vi "IRISS V2 Teleoperation.vi"() -> ()   [LabVIEW 2016]
uses:
  <vilib>/Math Plots/3D Math Plots/3D Scatter/3D Scatter XCtrl/3D Scatter.xctl
  <vilib>/Analysis/Matrix/Datatypes/RealMatrix.ctl
  Subsystems/Global Variables.vi
  <vilib>/Utility/file.llb/Read Delimited Spreadsheet (DBL).vi
  <vilib>/Math Plots/3D Math Plots/3D Scatter/3D Scatter Datatype/Public/Plot Helper (Vector).vi
  Library/mjglib/var_OCTzHomeDir.vi
  <vilib>/Math Plots/3D Math Plots/3D Plot/3D Plot Datatype/3D Plot Datatype.lvclass
  <vilib>/Analysis/Matrix/NI_Matrix.lvlib
  Functions/EyeRobotDLL.dll
  Library/KevinLibraryAll/labview2011/kevLib2011.lvlib
  <vilib>/Math Plots/3D Math Plots/3D Scatter/3D Scatter Datatype/3D Scatter Datatype.lvclass
panel:
  in  "MS/Auto":bool
  in  "Calib Params?":bool
  in  "Incision":bool caption="To M/S"
  in  "OCT Z PID Gains":cluster{"Kp":dbl, "Kd":dbl, "Ki":dbl}={"Kp"=0.0003, "Kd"=0.0001, "Ki"=0.01}
  out "deltaRoll":sgl
  out "deltaXYZ":sgl[](array[numeric])
  in  "To Regulation":bool
  in  "IRISS GUI":T1(tab)
  in  "U/S Power [%]":sgl min=0 max=100 step=10
  in  "Vac Cmd [mmHg]":sgl min=0 max=600 step=50
  in  "Red Round Box":u32(colorbox)=16711690
  in  "Blue Round Box":u32(colorbox)=16860
  in  "Black Round Box":u32(colorbox)
  out "Vacuum Force [mmHg]  2":i32 caption="[mmHg]"
  in  "IV Height [mmHg]":dbl=30.0 min=0.0 max=90.0 step=10.0
  in  "Irrigation":bool
  in  "Reroute Hold [sec]":dbl=10.0 caption="Hold [sec]"
  in  "Refractive Index":dbl=1.35
  out "Asgn Pt Out of Bound":bool caption="Assign Pt OOB"
  out "Emergency alarm":bool
  out "Remote sender engaged":bool
  out "State changing":bool
  out "Current Run No.":u8
  out "Tip out Posit":dbl[](array[numeric]) caption="Position [mm]" format="%#.3f"
  out "Tip cmd Posit":dbl[](array[numeric]) caption="Command [mm]" format="%#.3f"
  out "State Flag Array":bool[](array[boolean])
  out "Timer":i32 format="%<%M:%S>t"
  in  "Go to Assign Pt":bool
  out "Irrigation Engaged?":bool caption="Irrigation Engaged"
  out "Robot XYZ":refnum<class "3D Plot Datatype.lvclass">[](xcontrol)
  out "Current System State":T2(ring)
  in  "Tracking Mode":u16(ring) items=["Joint Mode", "XYZ Mode"]
  in  "Stage Z [mm]":dbl=100.0 min=-120.0 max=120.0 step=0.5
  in  "Stage Y [mm]":dbl=70.0 min=-120.0 max=100.0 step=0.5
  in  "Gripper":dbl
  in  "OCT Cmd Z [mm]":dbl min=-25.0 max=14.0 step=0.5
  out "Joint Out":dbl[](array[numeric])
  out "Robot Status Array":bool[](array[boolean])
  in  "L1 [deg]":dbl=-40.0
  in  "L2 [deg]":dbl=15.0
  in  "L3 [mm]":dbl=-5.0 step=0.1
  out "Status 2":bool[](array[boolean])
  in  "L4 [deg]":dbl=-10.0 step=0.1
  in  "Home":bool
  out "OCT Z out [mm]":dbl caption="OCT Out Z [mm]" format="%#.4f"
  in  "Tool Type":i32=6
  in  "Tool Offset [mm]":dbl=-50.68
  out "Grasp out":dbl format="%#.4g"
  in  "OCTz Home Dir":bool
  in  "Remote Control Source":u16(ring) caption="Remote Source" items=["None", "Surgical Console", "Joystick", "Rigid Joystick", "Zeiss PC", "MJG C++ Teleoperation", "A-Scan", ""]
  in  "Reset Joystick":bool caption="Encoder Reset"
  out "Send Count":u64
  out "Receive Count":u64
  out "Arm ID Ind":i32
  out "Status":bool
  in  "Stage X [mm]":dbl=30.0 min=-120.0 max=120.0 step=0.5
  out "XYZ Stage out":dbl[](array[numeric])
  out "XYZ Stage cmd":dbl[](array[numeric])
  out "DH Params":cluster{"d_DH":dbl[][], "ty":dbl[][]}
  in  "Eye No":i16=1 min=1 step=1
  in  "Reroute Transit Vacf":dbl=100.0
  in  "Z Rot Axis":dbl=1.0
  in  "Z Dist Thld":dbl[](array[numeric])=[3.0, 5.0] caption="Z Distance Threshould"
  in  "Vac Extremum":dbl[](array[numeric])=[68.0, 68.0] caption="Vacuum Extremum"
  out "Value [mmHg]":i8
  in  "Save Data":bool
  out "File Exists":bool
  out "File Path":path
  out "Elaspsed Time [s]":sgl
  in  "Data No":i16=1 min=1 step=1
  in  "Total Time":i16=90 min=1 step=1
  in  "Min PC Gap":dbl=0.1 caption="Min PC Gap [mm]" min=0.0 max=10.0 step=0.1 format="%#.3g"
  in  "Min AC Gap":dbl=0.1 caption="Min AC Gap [mm]" min=0.0 max=10.0 step=0.1 format="%#.3g"
  in  "Joint Limits":dbl[][](array[numeric])=[[-68.0, -4.0], [-26.0, 52.0], [-40.0, 23.0], [-180.0, 180.0]] format="%#.3g"
  out "L4 Waveform Graph":dbl[](graph)
  out "L3 Waveform Graph":dbl[](graph)
  out "L2 Waveform Graph":dbl[](graph)
  out "L1 Waveform Graph":dbl[](graph)
  in  "Inc Ctrl":dbl[](array[numeric])=[0.1, 0.05, 0.05] caption="Increment Control"
  out "Stage command":dbl[](array[numeric])
  in  "Vscan path":path=path "D:/IRISSoft LV2016 beta/Host Demo/ThorlabsData/Eye1/VSCAN_0002.raw"
  in  "size_xyz_mm":dbl[](array[numeric])=[16.0, 16.0, 9.4, 1.0]
  in  "size_xyz":dbl[](array[numeric])=[400.0, 400.0, 1024.0, 1.0]
  in  "Confirm":bool
  in  "Image index":i32=200
  out "O":dbl[](array[numeric])
  out "New TOI":dbl[][](array[numeric])
  out "Original TOI":dbl[][](array[numeric])
  in  "Stop Accurus":bool caption="To M/S"
  in  "L3 Go Home":bool caption="To M/S"
  in  "Program Stop":bool
  # "M/S\n \nAuto"
  # "Tool Tip Location"
  # "Tracking Planning"
  # "RCM"
  # "X\nY\nZ"
  # "X\nY\nZ"
  # "Tool"
  # "Trajectory"
  # "System Progress"
  # "Assign Point Rerouting"
  # "Trajectory Generation"
  # "X\nY\nZ"
  # "X Offset"
  # "Y Offset"
  # "Homing finished"
  # "Z Offset"
  # "M/S initialization finished"
  # "Tool Cruising Boundaries"
  # "XY-plane"
  # "Trajecoty loading finished"
  # "Aiming finished"
  # "Tool engaged"
  # "Z-axis"
  # "Phaco Machine"
  # "Tracking initialization finished"
  # "In Tracking"
  # "Rerouting finished"
  # "X\nY"
  # "X\nY"
  # "In regulation"
  # "Robot Control"
  # "Homing"
  # "Joint Definition"
  # "Arm"
  # "Tool"
  # "Stage"
  # "Robot Status"
  # "Joint M/S Cmd"
  # "HARDWARE_NOT_PRESENT"
  # "HARDWARE_NOT_FOUND_ALL_DRIVES"
  # "HARDWARE_SENSOR_FAULT"
  # "NOT_RUNNING"
  # "COMMUNICATION_ERROR"
  # "KINEMATICS_NO_SOLUTION"
  # "OCT Control"
  # "KINEMATICS_INSERTION_LENGTH_TOO_SMALL"
  # "COMMAND_BEYOND_JOINT_RANGE"
  # "COMMAND_TOO_LARGE"
  # "Irrigation and Aspiration"
  # "IOP Control"
  # "Data Saving"
  # "Irrigation"
  # "Aspiration"
  # "ACh"
  # "Vitreous"
  # "Rotation & Vacuum Force Scheduling"
  # "Joint Motion & Control"
  # "Space Deform Parameters"
  # "Depth Ctrl"
  # "S"
  # "R"
  # "[deg]"
  # "T"
  # "[mm]"
  # "First Track Point"
  # "AC & PC Gap"
  # "X1"
  # "[mm]"
  # "Y"
  # "[mm]"
  # "Z"
  # "[mm]"
  # "L4"
  # "[deg]"
  # "Joint Limits"
  # "Error Message"
  # "Incision"
  # "Min."
  # "Max."
  # "L1"
  # "[deg]"
  # "L1"
  # "L2"
  # "L2"
  # "[deg]"
  # "L3"
  # "[mm]"
  # "L3"
  # "L4"
  # "[deg]"
  # "L4"
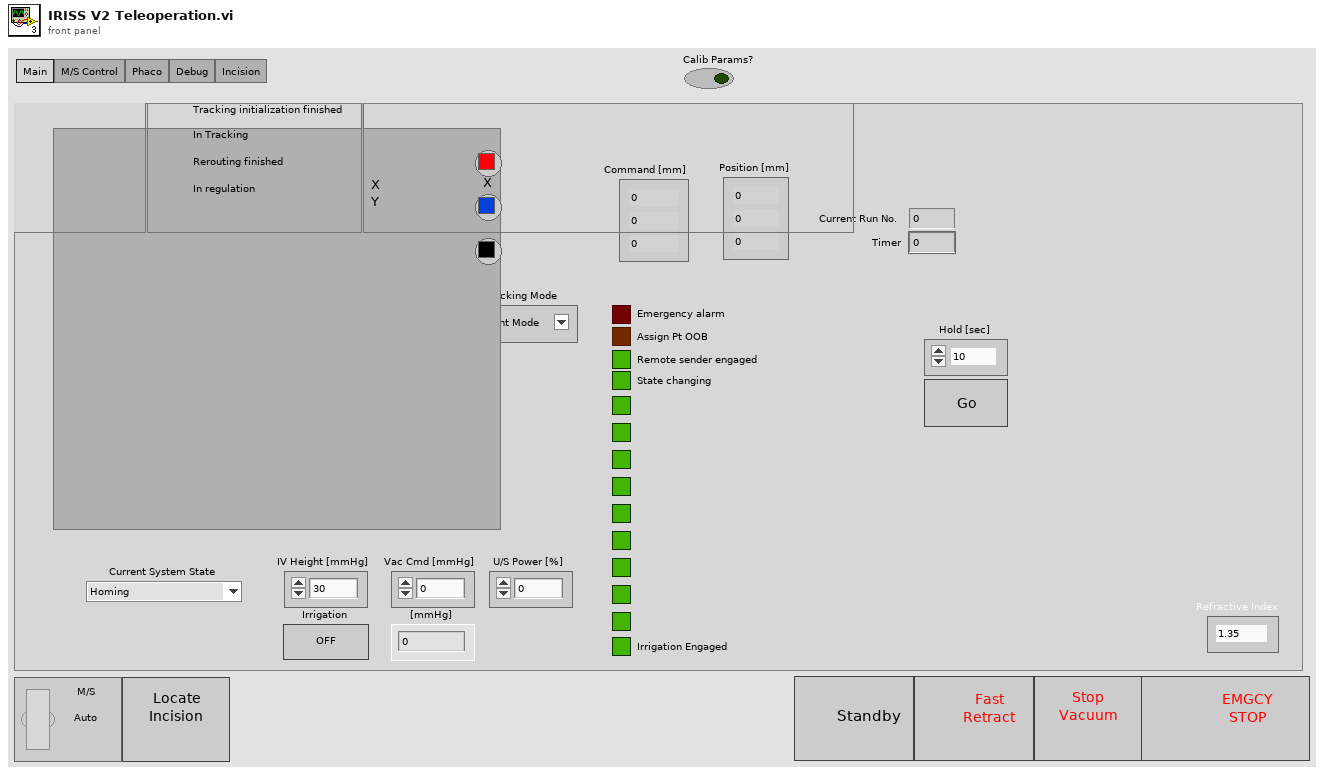
[diagram p1: front panel]
types:
  T1 = enum32{"Main", "M/S Control", "Phaco", "Debug", "Incision"}
  T2 = enum16{"Homing", "M/S Initialization", "M/S Operation", "Aiming", "Engaging", "Trajectory Loading", "Tracking Initialization", "Tracking", "Rerouting", "Regulation"}
  T3 = cluster{"Traj Px Array":dbl[], "Traj Py Array":dbl[], "Traj Pz Array":dbl[], "Speed Array":dbl[], "Depth Array":dbl[], "Traj Joint1 Array":dbl[], "Traj Joint2 Array":dbl[], "Traj Joint3 Array":dbl[], "Traj Joint4 Array":dbl[], "Traj Joint5 Array":dbl[]}
  T4 = typedef "NI_Matrix.lvlib/RealMatrix.ctl" = dbl[][]
  T5 = cluster{"X Grid":dbl[], "Y Grid":dbl[], "Za_true Surf":dbl[][], "Iris Center":dbl[], "Zp_true Surf":dbl[][], "Pinv":T4, "za_true":dbl, "za_work":dbl, "zp_work":dbl, "zp_true":dbl}
  T6 = enum8{"Enabled", "Disabled", "Disabled and Grayed Out"}
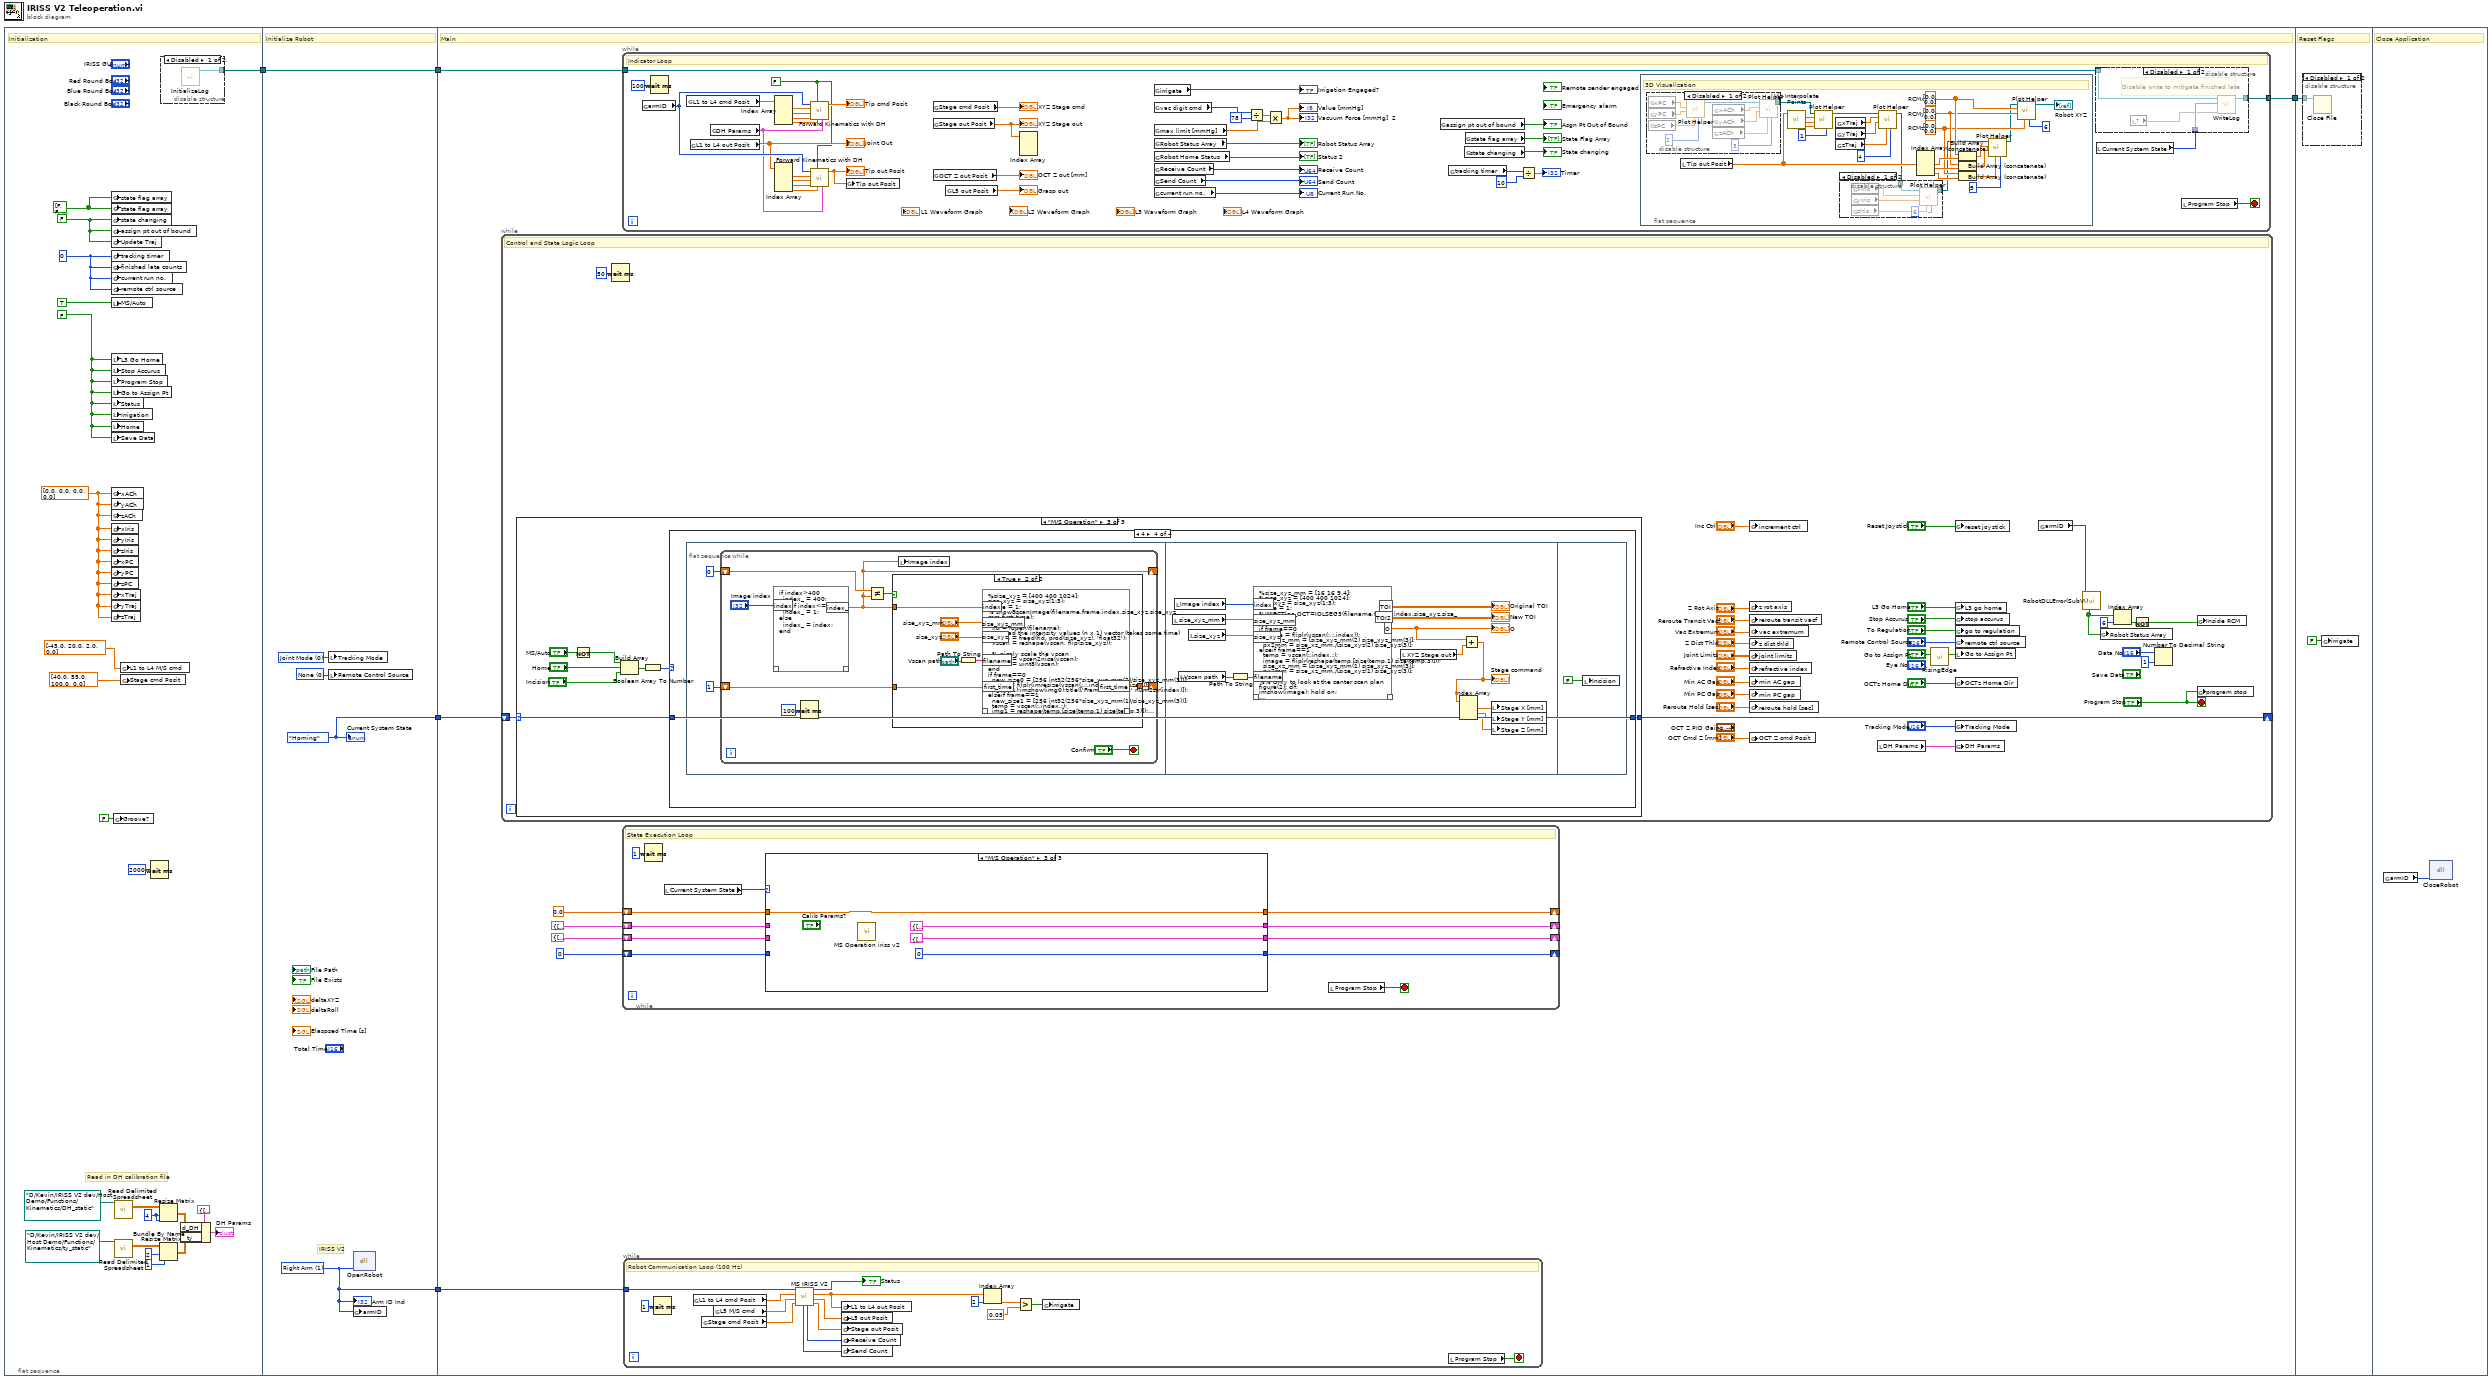
[diagram p0: block diagram]
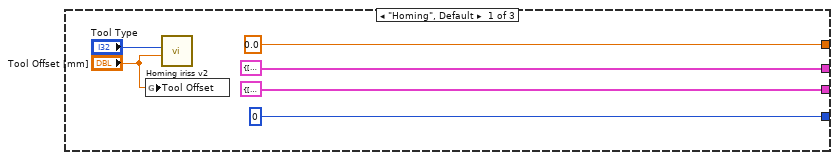
[diagram p3: hidden frame]
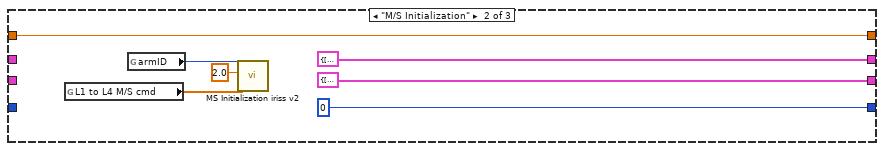
[diagram p4: hidden frame]
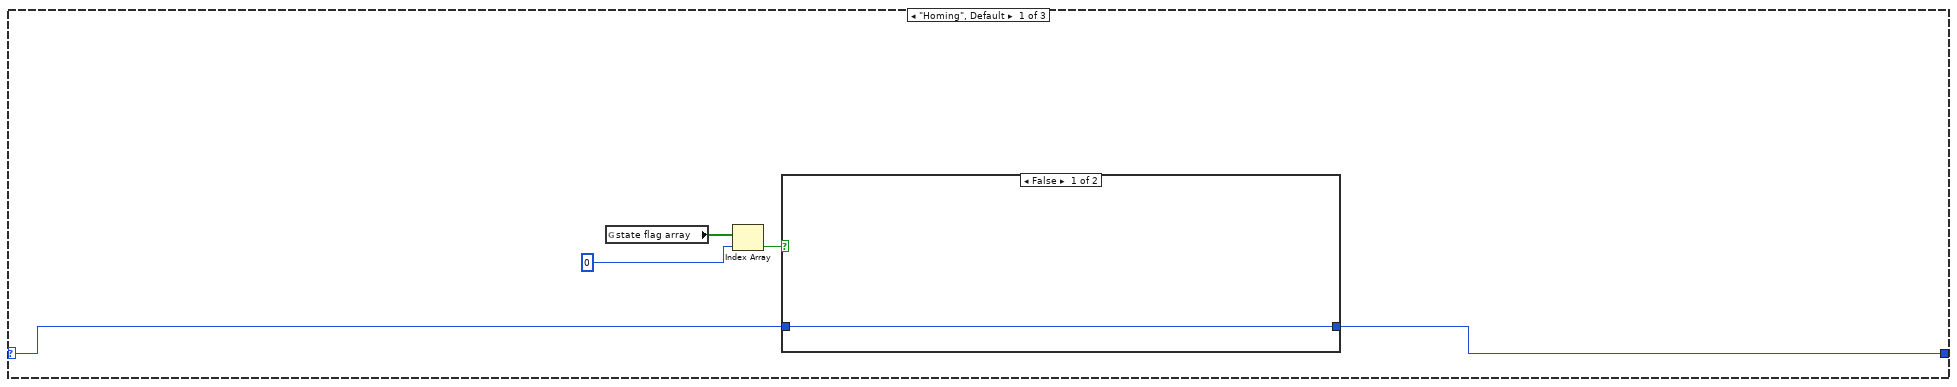
[diagram p8: hidden frame]
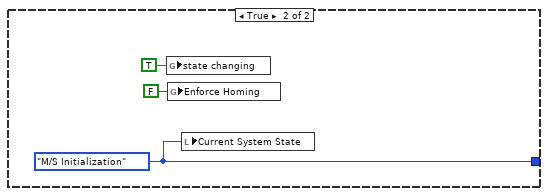
[diagram p9: hidden frame]
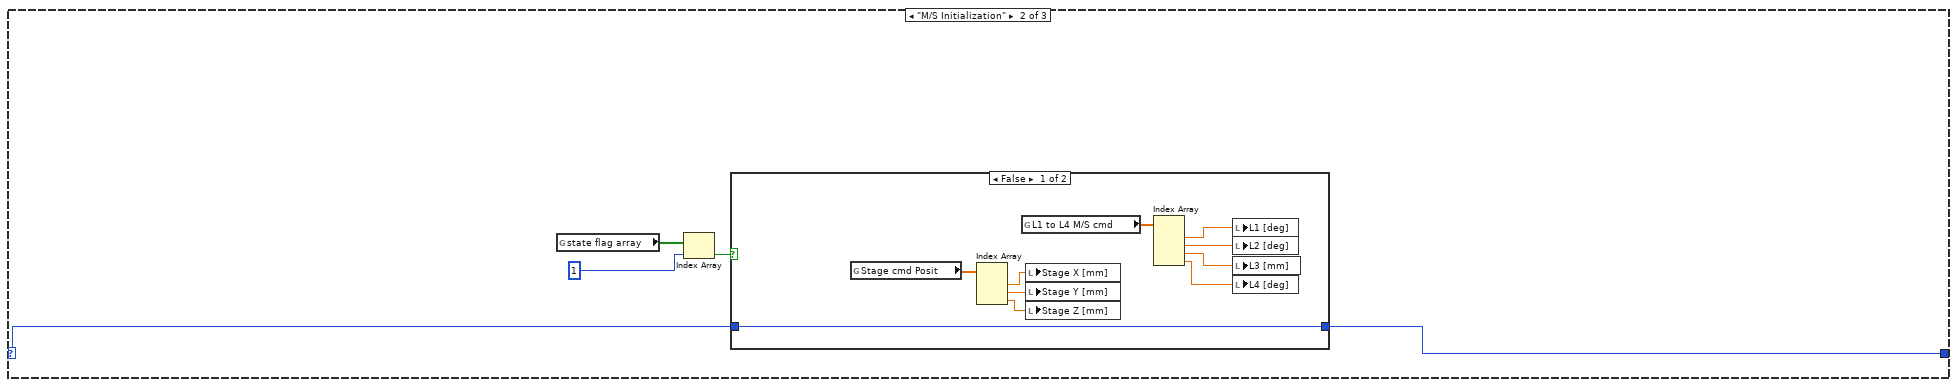
[diagram p10: hidden frame]
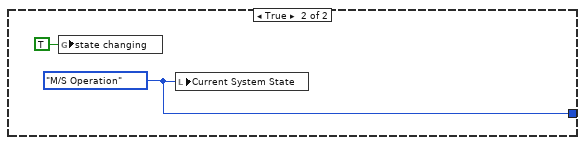
[diagram p11: hidden frame]
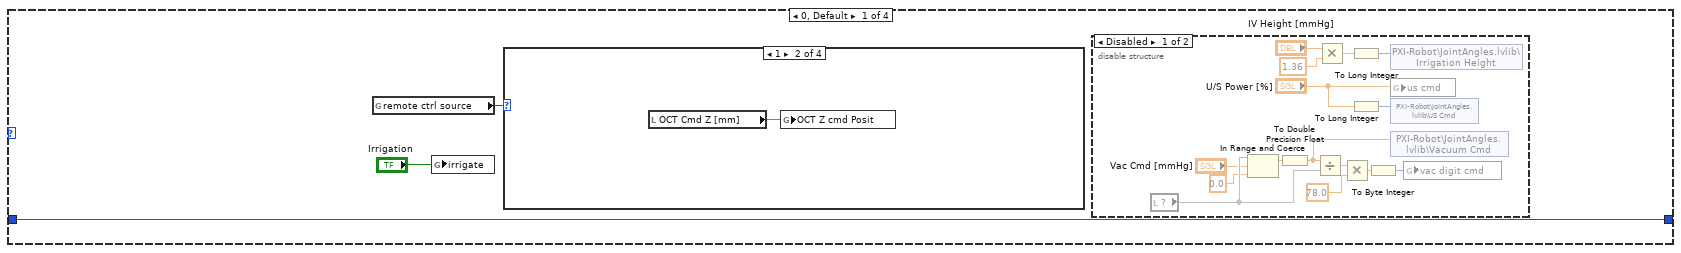
[diagram p12: hidden frame]
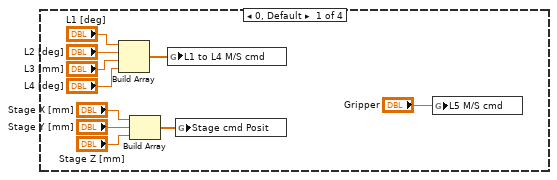
[diagram p14: hidden frame]
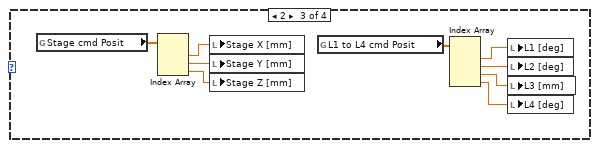
[diagram p15: hidden frame]
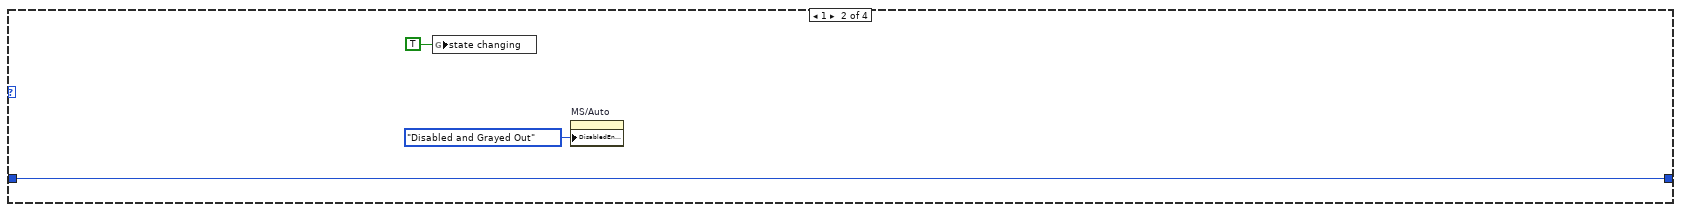
[diagram p17: hidden frame]
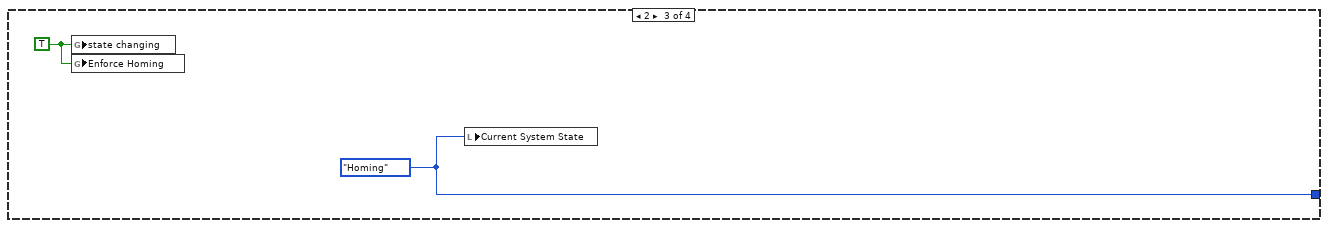
[diagram p18: hidden frame]
diagram:
  n1 = flat-sequence {
    tunnel: [w26] -> w3
    tunnel: [w32] -> w4
    tunnel: w3 -> [w33]
    tunnel: [w33] -> w2
    tunnel: [w30] -> w1
    tunnel: w4 -> [w41]
    tunnel: w2 -> [w40]
    tunnel: [w39] -> w5
    tunnel: w1 -> [w36]
    tunnel: w5 -> [w317]
    frame #0 {
      w14 = 4 ("number of rows")
      w21 = dbl[] [0.0, 0.0, 0.0, 0.0] ("First Trk Pt 2")
      w20 = 0 ("finished late counts")
      w25 = bool[] [FALSE, FALSE, FALSE, FALSE, FALSE, FALSE, FALSE, FALSE, FALSE] ("state flag array")
      w24 = FALSE ("state changing")
      w22 = FALSE ("program stop")
      # "Read in DH calibration file"
      # "Initialization"
      n2 = global write "Global Variables.vi" "state flag array"(w25) -> ()
      n3 = global write "Global Variables.vi" "state flag array"(w25) -> ()
      n4 = global write "Global Variables.vi" "state changing"(w24) -> ()
      n5 = global write "Global Variables.vi" "assign pt out of bound"(w24) -> ()
      n6 = global write "Global Variables.vi" "Update Traj"(w24) -> ()
      n7 = global write "Global Variables.vi" "tracking timer"(w20) -> ()
      n8 = global write "Global Variables.vi" "finished late counts"(w20) -> ()
      n9 = global write "Global Variables.vi" "current run no."(w20) -> ()
      n10 = global write "Global Variables.vi" "remote ctrl source"(w20) -> ()
      n11 = local write "MS/Auto"(TRUE ("MS/Auto")) -> ()
      n12 = local write "L3 Go Home"(w22) -> ()
      n13 = local write "Stop Accurus"(w22) -> ()
      n14 = local write "Program Stop"(w22) -> ()
      n15 = local write "Go to Assign Pt"(w22) -> ()
      n16 = local write "Status"(w22) -> ()
      n17 = local write "Irrigation"(w22) -> ()
      n18 = local write "Home"(w22) -> ()
      n19 = local write "Save Data"(w22) -> ()
      n20 = global write "Global Variables.vi" "xACh"(w21) -> ()
      n21 = global write "Global Variables.vi" "yACh"(w21) -> ()
      n22 = global write "Global Variables.vi" "zACh"(w21) -> ()
      n23 = global write "Global Variables.vi" "xIris"(w21) -> ()
      n24 = global write "Global Variables.vi" "yIris"(w21) -> ()
      n25 = global write "Global Variables.vi" "zIris"(w21) -> ()
      n26 = global write "Global Variables.vi" "xPC"(w21) -> ()
      n27 = global write "Global Variables.vi" "yPC"(w21) -> ()
      n28 = global write "Global Variables.vi" "zPC"(w21) -> ()
      n29 = global write "Global Variables.vi" "xTraj"(w21) -> ()
      n30 = global write "Global Variables.vi" "yTraj"(w21) -> ()
      n31 = global write "Global Variables.vi" "zTraj"(w21) -> ()
      n32 = global write "Global Variables.vi" "Groove?"(FALSE ("Groove?")) -> ()
      n33 = call-poly <vilib>:"Read Delimited Spreadsheet.vi"("file path (dialog if empty)"=path "D:/Kevin/IRISS V2 dev/Host Demo/Functions/Kinematics/DH_static" ("file path (use dialog)")) -> ("all rows"=w15:dbl[][])  [unwired: 9 in, 5 out]
      n34 = call-poly <vilib>:"Read Delimited Spreadsheet.vi"("file path (dialog if empty)"=path "D:/Kevin/IRISS V2 dev/Host Demo/Functions/Kinematics/ty_static" ("file path (use dialog)")) -> ("all rows"=w13:dbl[][])  [unwired: 9 in, 5 out]
      n35 = global write "Global Variables.vi" "L1 to L4 M/S cmd"(dbl[] [-45.0, 20.0, 2.0, 0.0] ("First Trk Pt 2")) -> ()
      n36 = global write "Global Variables.vi" "Stage cmd Posit"(dbl[] [40.0, 55.0, 100.0, 0.0] ("First Trk Pt 2")) -> ()
      n37 = Wait (ms)(milliseconds to wait=u32 2000) -> ()  [unwired: 1 out]
      n38 = Resize Matrix(1:w14, 2:w14, 4:w15) -> (0:w9:dbl[][])
      n39 = Resize Matrix(1:1 ("number of columns"), 2:2 ("number of rows"), 4:w13) -> (0:w8:dbl[][])
      n40 = disable-structure shown="Disabled" {
        disable-tunnel: [w28 _] -> w26
        frame Disabled {
          n41 = call "InitializeLog.vi"() -> ("Byte Stream File out"=w28:refnum<file>)  [unwired: 11 in]
        }
        frame Enabled {
        }
      }
      n42 = Bundle By Name(cluster=cluster{"d_DH":dbl[][], "ty":dbl[][]} {"d_DH"=[[0.0, -0.04858099004841317, 1.1971672750675049, 0.0], [0.0, -1.576475511297109, 0.0, 0.0], [-0.3552491783526254, 0.0, -1.1064589410656984, 0.2058446720735121], [-1.0573457532495087, 1.0278049025155533, 0.011917110633363169, -0.004023577880993236]], "ty"=[[0.04320445582455471], [0.011728642746432275]]} ("input cluster"), "d_DH"=w9, "ty"=w8) -> (→"DH Params":cluster{"d_DH":dbl[][], "ty":dbl[][]})
    }
    frame #1 {
      w29 = u16 0 items=["Joint Mode", "XYZ Mode"] ("Tracking Mode")
      w31 = u16 0 items=["None", "Surgical Console", "Joystick", "MJG Teleoperation", "MJG C++ Teleoperation"] ("Remote Control Source 2")
      w32 = T2."Homing" ("Current State")
      w30 = 1 items=["Left Arm", "Right Arm"] ("Left or Right Arm")
      # "IRISS V2"
      # "Initialize Robot"
      n43 = local write "Tracking Mode"(w29) -> ()
      n44 = local write "Remote Control Source"(w31) -> ()
      n45 = dll-call lib="D:/Kevin/IRISS V2 dev/Host Demo/Functions/EyeRobotDLL.dll" fn="OpenRobot" label="Open"("id"=w30) -> ()  [unwired: 5 in, 2 out]
      n46 = global write "Global Variables.vi" "armID"(w30) -> ()
      "Arm ID Ind" <- w30
      "Current System State" <- w32
    }
    frame #2 {
      # "Main"
      n47 = while {
        shift-right: [w195] -> _
        shift-left: w41 -> [w196]
        stop <- "Program Stop" stop-if-true
        # "Control and State Logic Loop"
        n48 = case shown="\"M/S Operation\"" w196 {
          selector: w196 -> [w208 w215 w239]
          tunnel: [w207 w216 w238] -> w195
          frame "Homing", Default {
            # "State Diagram"
            n49 = global read "Global Variables.vi" "state flag array"() -> (w209:bool[])
            n50 = Index Array(array=w209, index=0) -> (element=w206:bool)
            n51 = case shown="False" w206 {
              tunnel: [w211 w213] -> w207
              tunnel: w208 -> [w211 _]
              frame False {
                # "homing in process"
              }
              frame True {
                w213 = T2."M/S Initialization" ("Current State")
                # "finish homing"
                n52 = global write "Global Variables.vi" "state changing"(TRUE ("state changing")) -> ()
                n53 = global write "Global Variables.vi" "Enforce Homing"(FALSE ("Enforce Homing")) -> ()
                n54 = local write "Current System State"(w213) -> ()
              }
            }
          }
          frame "M/S Initialization" {
            n55 = global read "Global Variables.vi" "state flag array"() -> (w218:bool[])
            n56 = Index Array(array=w218, index=1) -> (element=w217:bool)
            n57 = case shown="False" w217 {
              tunnel: [w229 w230] -> w216
              tunnel: w215 -> [w229 _]
              frame False {
                n58 = global read "Global Variables.vi" "Stage cmd Posit"() -> (w223:dbl[])
                n59 = Index Array(array=w223) -> (element #1=w221:dbl, element #2=w222:dbl, element #3=w220:dbl)  [unwired: 3 in]
                n60 = global read "Global Variables.vi" "L1 to L4 M/S cmd"() -> (w228:dbl[])
                n61 = local write "Stage X [mm]"(w221) -> ()
                n62 = local write "Stage Y [mm]"(w222) -> ()
                n63 = local write "Stage Z [mm]"(w220) -> ()
                n64 = Index Array(array=w228) -> (element #1=w227:dbl, element #2=w226:dbl, element #3=w225:dbl, element #4=w224:dbl)  [unwired: 4 in]
                n65 = local write "L1 [deg]"(w227) -> ()
                n66 = local write "L2 [deg]"(w226) -> ()
                n67 = local write "L3 [mm]"(w225) -> ()
                n68 = local write "L4 [deg]"(w224) -> ()
              }
              frame True {
                w230 = T2."M/S Operation" ("Current State")
                n69 = global write "Global Variables.vi" "state changing"(TRUE ("state changing")) -> ()
                n70 = local write "Current System State"(w230) -> ()
              }
            }
          }
          frame "M/S Operation" {
            n71 = Not(x="MS/Auto") -> (.not. x?=w237:bool)
            n72 = Build Array(w237, "Home", "Incision") -> (w236:bool[])
            n73 = Boolean Array To Number(Boolean array=w236) -> (number=w235:u32)
            n74 = case shown="4" w235 {
              tunnel: w239 -> [w242 w279 _ w283]
              tunnel: [w242 w279 w282 w283] -> w238
              frame 0, Default {
                n75 = global read "Global Variables.vi" "remote ctrl source"() -> (w241:u16)
                n76 = global write "Global Variables.vi" "irrigate"("Irrigation") -> ()
                n77 = case shown="1" w241 {
                  frame 0, Default {
                    n78 = Build Array("L1 [deg]", "L2 [deg]", "L3 [mm]", "L4 [deg]") -> (w258:dbl[])
                    n79 = Build Array("Stage X [mm]", "Stage Y [mm]", "Stage Z [mm]") -> (w263:dbl[])
                    n80 = global write "Global Variables.vi" "L1 to L4 M/S cmd"(w258) -> ()
                    n81 = global write "Global Variables.vi" "Stage cmd Posit"(w263) -> ()
                    n82 = global write "Global Variables.vi" "L5 M/S cmd"("Gripper") -> ()
                  }
                  frame 1 {
                    n83 = local read "OCT Cmd Z [mm]"() -> (w268:dbl)
                    n84 = global write "Global Variables.vi" "OCT Z cmd Posit"(w268) -> ()
                  }
                  frame 2 {
                    n85 = global read "Global Variables.vi" "Stage cmd Posit"() -> (w277:dbl[])
                    n86 = Index Array(array=w277) -> (element #1=w276:dbl, element #2=w275:dbl, element #3=w274:dbl)  [unwired: 3 in]
                    n87 = local write "Stage X [mm]"(w276) -> ()
                    n88 = local write "Stage Y [mm]"(w275) -> ()
                    n89 = local write "Stage Z [mm]"(w274) -> ()
                    n90 = global read "Global Variables.vi" "L1 to L4 cmd Posit"() -> (w269:dbl[])
                    n91 = Index Array(array=w269) -> (element #1=w272:dbl, element #2=w271:dbl, element #3=w270:dbl, element #4=w273:dbl)  [unwired: 4 in]
                    n92 = local write "L1 [deg]"(w272) -> ()
                    n93 = local write "L2 [deg]"(w271) -> ()
                    n94 = local write "L3 [mm]"(w270) -> ()
                    n95 = local write "L4 [deg]"(w273) -> ()
                  }
                  frame 3 {
                  }
                }
                n96 = disable-structure shown="Disabled" {
                  frame Disabled {
                    n97 = local read item#-1() -> (w249)
                    n98 = In Range and Coerce(upper limit=w249, x="Vac Cmd [mmHg]", lower limit=0.0) -> (coerced(x)=w250:dbl)  [unwired: 1 out]
                    n99 = To Double Precision Float(number=w250) -> (double precision float=w251:dbl)
                    n100 = Divide(x=w251, y=w249) -> (x/y=w244:dbl)
                    n101 = Multiply(x="IV Height [mmHg]", y=1.36) -> (x*y=w255:dbl)
                    n102 = Multiply(x=w244, y=78.0) -> (x*y=w246:dbl)
                    n103 = To Long Integer(number=w255) -> (32bit integer=w256:i32)
                    n104 = To Long Integer(number="U/S Power [%]") -> (32bit integer=w252:i32)
                    n105 = To Byte Integer(number=w246) -> (8bit integer=w243:i8)
                    n106 = shared-variable "PXI-Robot\\JointAngles.lvlib\\Irrigation Height"(w256) -> ()  [unwired: 1 in, 1 out]
                    n107 = global write "Global Variables.vi" "us cmd"("U/S Power [%]") -> ()
                    n108 = shared-variable "PXI-Robot\\JointAngles.lvlib\\US Cmd"(w252) -> ()  [unwired: 1 in, 1 out]
                    n109 = shared-variable "PXI-Robot\\JointAngles.lvlib\\Vacuum Cmd"(w251) -> ()  [unwired: 1 in, 1 out]
                    n110 = global write "Global Variables.vi" "vac digit cmd"(w243) -> ()
                  }
                  frame Enabled {
                  }
                }
              }
              frame 1 {
                n111 = global write "Global Variables.vi" "state changing"(TRUE ("state changing")) -> ()
                n112 = property on="MS/Auto" class="Bool (strict)"("DisabledEnum"=T6."Disabled and Grayed Out" ("Disabled")) -> ()  [unwired: 2 in, 2 out]
              }
              frame 2 {
                w282 = T2."Homing" ("Current State")
                w281 = TRUE ("state changing")
                n113 = global write "Global Variables.vi" "state changing"(w281) -> ()
                n114 = global write "Global Variables.vi" "Enforce Homing"(w281) -> ()
                n115 = local write "Current System State"(w282) -> ()
              }
              frame 4 {
                n116 = flat-sequence {
                  frame #0 {
                    n117 = while {
                      shift-right: [w290] -> _
                      shift-left: 0 -> [w291]
                      shift-right: [w288] -> _
                      shift-left: 1 -> [w289]
                      stop <- "Confirm" stop-if-true
                      n118 = script code="if index>400\n  index_ = 400;\nelseif index<=0\n  index_ = 1;\nelse\n  index_ = index;\nend"("index"="Image index") -> ("index_"=w290:dbl)  [unwired: 1 in, 1 out]
                      n119 = Wait (ms)(milliseconds to wait=u32 100) -> ()  [unwired: 1 out]
                      n120 = Not Equal?(x=w291, y=w290) -> (x != y?=w292:bool)
                      n121 = case shown="True" w292 {
                        tunnel: w290 -> [_ w301]
                        tunnel: w289 -> [w294 w299]
                        tunnel: [w294 w298] -> w288
                        frame False {
                        }
                        frame True {
                          n122 = Path To String(path="Vscan path") -> (string=w300:string)
                          n123 = script code="%size_xyz = [400 400 1024];\nsize_xyz = size_xyz(1:3);\nframe = 1;\n% showBscanImage(filename,frame,index,size_xyz,size_xyz_mm,first_time);\nif first_time\n  fid = fopen(filename);\n  % Read the intensity values (n x 1) vector (takes some time)\n  vscan = fread(fid, prod(size_xyz), 'float32');\n  vscan = reshape(vscan, flip(size_xyz));\n\n  % nicely scale the vscan\n  vscan = vscan2nice(vscan);\n  vscan = uint8(vscan);\nend\nif frame==0\n  new_size0 = [256 int32(256*size_xyz_mm(2)/size_xyz_mm(3))];\n  img0 = filplr(imresize(vscan(:,:,index),new_size0));\n  figure(1);imshow(img0);title(['Frame:0 Index:' num2str(index)]);\nelseif frame==1\n  new_size1 = [256 int32(256*size_xyz_mm(1)/size_xyz_mm(3))];\n  temp = vscan(:,index,:);\n  img1 = reshape(temp,[size(temp,1) size(temp,3)]);\n  img1 = fliplr(imresize(img1,new_size1));\n  figure(1);imshow(img1);title(['Frame:1 Index:' num2str(index)]);\nend\n\nfirst_time = 0;"("index"=w301, "size_xyz_mm"="size_xyz_mm", "size_xyz"="size_xyz", "filename"=w300, "first_time"=w299) -> ("first_time"=w298:dbl)  [unwired: 1 in, 1 out]
                        }
                      }
                      n124 = local write "Image index"(w290) -> ()
                    }
                  }
                  frame #1 {
                    n125 = local read "size_xyz_mm"() -> (w313:dbl[])
                    n126 = local read "Image index"() -> (w314:i32)
                    n127 = local read "Vscan path"() -> (w311:path)
                    n128 = local read "size_xyz"() -> (w312:dbl[])
                    n129 = Path To String(path=w311) -> (string=w310:string)
                    n130 = script code="%size_xyz_mm = [16 16 9.4];\n%size_xyz = [400 400 1024];\nsize_xyz = size_xyz(1:3);\nframe = 1;\n%INJECTloc_OCT=IOLSEG3(filename,frame,index,size_xyz,size_xyz_mm);\n\nif frame==0\n  image = fliplr(vscan(:,:,index));\n  size_xz_mm = [size_xyz_mm(2) size_xyz_mm(3)];\n  px2mm = size_xz_mm./[size_xyz(2) size_xyz(3)]; \nelseif frame==1\n  temp = vscan(:,index,:);\n  image = fliplr(reshape(temp,[size(temp,1) size(temp,3)]));\n  size_xz_mm = [size_xyz_mm(1) size_xyz_mm(3)];\n  px2mm = size_xz_mm./[size_xyz(1) size_xyz(3)]; \nend\n%% Only to look at the center scan plan\nfigure(2); clf; \nimshow(image); hold on;\n    \n% Collect two user clicks of Injection location \n[input1, Zinput1] = ginput(1);\nplot(input1, Zinput1, 'rx', 'MarkerSize', 20, 'LineWidth', 3); \n[input2, Zinput2] = ginput(1); % Collect two user clicks \nplot(input2, Zinput2, 'rx', 'MarkerSize', 20, 'LineWidth', 3); \n    \nYinput1 = size_xyz(2) - input1; \nYinput2 = size_xyz(2) - input2;\n    \nINJECTloc_px = [Yinput1, Zinput1; ... \n        Yinput2, Zinput2]; % [px] \nINJECTloc_px_mid=[(INJECTloc_px(1,1)+INJECTloc_px(2,1))/2,(INJECTloc_px(2,1)+INJECTloc_px(2,2))/2];\nclose(2); % close figure\n    \n% Convert these two locations from pixels to {OCT} frame  \nxloc_OCT = index/400*size_xz_mm(1); % B-scan is halfway through the image\nINJECTloc_OCT = [xloc_OCT*ones(1,1), INJECTloc_px_mid(1,1)*px2mm(1),  INJECTloc_px_mid(1,2)*px2mm(2)];\n\nincision_pt = [INJECTloc_OCT(1:3),1]';\nTOI_file= 'D:\\IRISSoft LV2016 beta\\Host Demo\\TOI_static'\nfid_TOI = fopen(TOI_file,'r');\nTOI=fscanf(fid_TOI,'%f');\nTOI= reshape(TOI, [4 4])';\nfclose(fid_TOI);\n\nO = inv(TOI)*incision_pt;\n%init_X = 40;init_Y = 55;init_Z = 100;\n%time_to_go = norm(O(1:3))/.5;\n%traj = [linspace(0,O(1),1000*time_to_go);linspace(0,O(2),1000*time_to_go);linspace(0,O(3),1000*time_to_go)];\n%stage_X = linspace(init_X,init_X+O(1),1000*time_to_go);\n%stage_Y = linspace(init_Y,init_Y+O(2),1000*time_to_go);\n%stage_Z = linspace(init_Z,init_Z+O(3),1000*time_to_go);\n\nTOI2 = inv(TOI);TOI2(1:3,4) = TOI2(1:3,4)-O(1:3);\nTOI2 = inv(TOI2);\nO = O';\n\nTOI2_file= 'D:\\IRISSoft LV2016 beta\\Host Demo\\new_TOI.txt';\nfid_TOI2 = fopen(TOI2_file,'w');\nfmt = [repmat('%.10f ', 1, 4), '\\n'];\nfprintf(fid_TOI2, fmt, TOI2');\nfclose(fid_TOI2);"("index"=w314, "size_xyz_mm"=w313, "size_xyz"=w312, "filename"=w310) -> ("TOI"=→"Original TOI":dbl[][], "TOI2"=→"New TOI":dbl[][], "O"=w307:dbl[])  [unwired: 1 in, 1 out]
                    "O" <- w307
                    n131 = local read "XYZ Stage out"() -> (w306:dbl[])
                    n132 = Add(x=w307, y=w306) -> (x+y=w305:dbl[])
                    "Stage command" <- w305
                    n133 = Index Array(array=w305) -> (element #1=w304:dbl, element #2=w303:dbl, element #3=w302:dbl)  [unwired: 3 in]
                    n134 = local write "Stage X [mm]"(w304) -> ()
                    n135 = local write "Stage Y [mm]"(w303) -> ()
                    n136 = local write "Stage Z [mm]"(w302) -> ()
                  }
                  frame #2 {
                    n137 = local write "Incision"(FALSE) -> ()
                  }
                }
              }
            }
          }
        }
        n138 = Wait (ms)(milliseconds to wait=u32 50) -> ()  [unwired: 1 out]
        n139 = global write "Global Variables.vi" "increment ctrl"("Inc Ctrl") -> ()
        n140 = global write "Global Variables.vi" "z rot axis"("Z Rot Axis") -> ()
        n141 = global write "Global Variables.vi" "reroute transit vacf"("Reroute Transit Vacf") -> ()
        n142 = global write "Global Variables.vi" "vac extremum"("Vac Extremum") -> ()
        n143 = global write "Global Variables.vi" "z dist thld"("Z Dist Thld") -> ()
        n144 = global write "Global Variables.vi" "joint limits"("Joint Limits") -> ()
        n145 = global write "Global Variables.vi" "refractive index"("Refractive Index") -> ()
        n146 = global write "Global Variables.vi" "min AC gap"("Min AC Gap") -> ()
        n147 = global write "Global Variables.vi" "min PC gap"("Min PC Gap") -> ()
        n148 = global write "Global Variables.vi" "reroute hold [sec]"("Reroute Hold [sec]") -> ()
        n149 = global write "Global Variables.vi" "OCT Z cmd Posit"("OCT Cmd Z [mm]") -> ()
        n150 = local read "DH Params"() -> (w174:cluster{"d_DH":dbl[][], "ty":dbl[][]})
        n151 = call "RisingEdge.vi"("Signal In"="Go to Assign Pt") -> ("Rising Edge"=w186:bool)  [unwired: 10 in]
        n152 = global write "Global Variables.vi" "reset joystick"("Reset Joystick") -> ()
        n153 = global write "Global Variables.vi" "L3 go home"("L3 Go Home") -> ()
        n154 = global write "Global Variables.vi" "stop accurus"("Stop Accurus") -> ()
        n155 = global write "Global Variables.vi" "go to regulation"("To Regulation") -> ()
        n156 = global write "Global Variables.vi" "remote ctrl source"("Remote Control Source") -> ()
        n157 = local write "Go to Assign Pt"(w186) -> ()
        n158 = global write "var_OCTzHomeDir.vi" "OCTz Home Dir"("OCTz Home Dir") -> ()
        n159 = global write "Global Variables.vi" "Tracking Mode"("Tracking Mode") -> ()
        n160 = global write "Global Variables.vi" "DH Params"(w174) -> ()
        n161 = global read "Global Variables.vi" "armID"() -> (w184:i32)
        n162 = call "RobotDLLError(SubVI).vi"("ArmID"=w184) -> ("RobotStatusArray"=w183:bool[])  [unwired: 5 in, 9 out]
        n163 = global write "Global Variables.vi" "Robot Status Array"(w183) -> ()
        n164 = Index Array(array=w183, index=6) -> (element=w181:bool)
        n165 = Not(x=w181) -> (.not. x?=w180:bool)
        n166 = Number To Decimal String(number="Data No", width (-)=i16 1) -> ()  [unwired: 1 out]
        n167 = global write "Global Variables.vi" "Inside RCM"(w180) -> ()
        n168 = global write "Global Variables.vi" "program stop"("Program Stop") -> ()
      }
      n169 = while {
        shift-right: [w66] -> _
        shift-left: 0.0 ("Prev OCT Z Posit") -> [w67]
        shift-right: [w64] -> _
        shift-left: 0 -> [w63]
        shift-right: [w62] -> _
        shift-left: T3 {"Traj Px Array"=[], "Traj Py Array"=[], "Traj Pz Array"=[], "Speed Array"=[], "Depth Array"=[], "Traj Joint1 Array"=[], "Traj Joint2 Array"=[], "Traj Joint3 Array"=[], "Traj Joint4 Array"=[], "Traj Joint5 Array"=[]} ("Trajectory Cluster 2") -> [w60]
        shift-right: [w61] -> _
        shift-left: T5 {"X Grid"=[], "Y Grid"=[], "Za_true Surf"=[], "Iris Center"=[0.0, 5.0, 0.0], "Zp_true Surf"=[], "Pinv"=[[1.0, 0.0], [0.0, 1.0]], "za_true"=0.0, "za_work"=0.0, "zp_work"=0.0, "zp_true"=0.0} ("Eye Model Cluster") -> [w59]
        stop <- w65 stop-if-true
        # "State Execution Loop"
        n170 = Wait (ms)(milliseconds to wait=u32 1) -> ()  [unwired: 1 out]
        n171 = local read "Current System State"() -> (w58:T2)
        n172 = case shown="\"M/S Operation\"" w58 {
          tunnel: w67 -> [_ w78 w82]
          tunnel: [0.0 ("Prev OCT Z Posit") w78 w82] -> w66
          tunnel: [0 ("Last Index") 0 ("Last Index") 0 ("Last Index")] -> w64
          tunnel: w63 -> [_ _ _]
          tunnel: [T3 {"Traj Px Array"=[], "Traj Py Array"=[], "Traj Pz Array"=[], "Speed Array"=[], "Depth Array"=[], "Traj Joint1 Array"=[], "Traj Joint2 Array"=[], "Traj Joint3 Array"=[], "Traj Joint4 Array"=[], "Traj Joint5 Array"=[]} ("Trajectory Cluster 2") T3 {"Traj Px Array"=[], "Traj Py Array"=[], "Traj Pz Array"=[], "Speed Array"=[], "Depth Array"=[], "Traj Joint1 Array"=[], "Traj Joint2 Array"=[], "Traj Joint3 Array"=[], "Traj Joint4 Array"=[], "Traj Joint5 Array"=[]} ("Trajectory Cluster 2") T3 {"Traj Px Array"=[], "Traj Py Array"=[], "Traj Pz Array"=[], "Speed Array"=[], "Depth Array"=[], "Traj Joint1 Array"=[], "Traj Joint2 Array"=[], "Traj Joint3 Array"=[], "Traj Joint4 Array"=[], "Traj Joint5 Array"=[]} ("Trajectory Cluster 2")] -> w62
          tunnel: [T5 {"X Grid"=[], "Y Grid"=[], "Za_true Surf"=[], "Iris Center"=[0.0, 5.0, 0.0], "Zp_true Surf"=[], "Pinv"=[[1.0, 0.0], [0.0, 1.0]], "za_true"=0.0, "za_work"=0.0, "zp_work"=0.0, "zp_true"=0.0} ("Eye Model Cluster") T5 {"X Grid"=[], "Y Grid"=[], "Za_true Surf"=[], "Iris Center"=[0.0, 5.0, 0.0], "Zp_true Surf"=[], "Pinv"=[[1.0, 0.0], [0.0, 1.0]], "za_true"=0.0, "za_work"=0.0, "zp_work"=0.0, "zp_true"=0.0} ("Eye Model Cluster") T5 {"X Grid"=[], "Y Grid"=[], "Za_true Surf"=[], "Iris Center"=[0.0, 5.0, 0.0], "Zp_true Surf"=[], "Pinv"=[[1.0, 0.0], [0.0, 1.0]], "za_true"=0.0, "za_work"=0.0, "zp_work"=0.0, "zp_true"=0.0} ("Eye Model Cluster")] -> w61
          tunnel: w60 -> [_ _ _]
          tunnel: w59 -> [_ _ _]
          frame "Homing", Default {
            n173 = global write "Global Variables.vi" "Tool Offset"("Tool Offset [mm]") -> ()
            n174 = call "Homing iriss v2.vi"("Tool Offset"="Tool Offset [mm]", "ToolType"="Tool Type") -> ()  [unwired: 10 in]
          }
          frame "M/S Initialization" {
            n175 = global read "Global Variables.vi" "L1 to L4 M/S cmd"() -> (w75:dbl[])
            n176 = global read "Global Variables.vi" "armID"() -> (w76:i32)
            n177 = call "MS Initialization iriss v2.vi"("Destination Posit Array [mm]"=w75, "Ramp Time [sec]"=2.0, "armID"=w76) -> ()  [unwired: 9 in]
          }
          frame "M/S Operation" {
            n178 = call "MS Operation iriss v2.vi"() -> ()  [unwired: 12 in]
          }
        }
        n179 = local read "Program Stop"() -> (w65:bool)
      }
      n180 = while {
        tunnel: w40 -> [w118]
        tunnel: [w117] -> w39
        stop <- w125 stop-if-true
        w86 = FALSE ("DH Calib?")
        # "Indicator Loop"
        n181 = global read "Global Variables.vi" "armID"() -> (w95:i32)
        n182 = Wait (ms)(milliseconds to wait=u32 100) -> ()  [unwired: 1 out]
        n183 = global read "Global Variables.vi" "L1 to L4 cmd Posit"() -> (w100:dbl[])
        n184 = global read "Global Variables.vi" "L1 to L4 out Posit"() -> (w94:dbl[])
        "Joint Out" <- w94
        n185 = global read "Global Variables.vi" "DH Params"() -> (w89:cluster{"d_DH":dbl[][], "ty":dbl[][]})
        n186 = Index Array(array=w100) -> (element #1=w99:dbl, element #2=w98:dbl, element #3=w97:dbl, element #4=w96:dbl)  [unwired: 4 in]
        n187 = Index Array(array=w94) -> (element #1=w93:dbl, element #2=w92:dbl, element #3=w91:dbl, element #4=w90:dbl)  [unwired: 4 in]
        n188 = call "Forward Kinematics with DH.vi"("DH Params"=w89, "j4"=w96, "DH Calib?"=w86, "j3"=w97, "j2"=w98, "j1"=w99, "armID"=w95) -> ("XYZ"=→"Tip cmd Posit":dbl[])  [unwired: 2 in, 2 out]
        n189 = call "Forward Kinematics with DH.vi"("DH Params"=w89, "j4"=w90, "DH Calib?"=w86, "j3"=w91, "j2"=w92, "j1"=w93, "armID"=w95) -> ("XYZ"=w87:dbl[])  [unwired: 2 in, 2 out]
        "Tip out Posit" <- w87
        n190 = global write "Global Variables.vi" "Tip out Posit"(w87) -> ()
        n191 = global read "Global Variables.vi" "Stage cmd Posit"() -> (→"XYZ Stage cmd":dbl[])
        n192 = global read "Global Variables.vi" "Stage out Posit"() -> (w103:dbl[])
        "XYZ Stage out" <- w103
        n193 = global read "Global Variables.vi" "OCT Z out Posit"() -> (→"OCT Z out [mm]":dbl)
        n194 = global read "Global Variables.vi" "L5 out Posit"() -> (→"Grasp out":dbl)
        n195 = Index Array(array=w103) -> ()  [unwired: 3 in, 3 out]
        n196 = global read "Global Variables.vi" "irrigate"() -> (→"Irrigation Engaged?":bool)
        n197 = global read "Global Variables.vi" "vac digit cmd"() -> (w108:i8)
        n198 = global read "Global Variables.vi" "max limit [mmHg]"() -> (w105:dbl)
        n199 = global read "Global Variables.vi" "Robot Status Array"() -> (→"Robot Status Array":bool[])
        n200 = global read "Global Variables.vi" "Robot Home Status"() -> (→"Status 2":bool[])
        n201 = global read "Global Variables.vi" "Receive Count"() -> (→"Receive Count":u64)
        n202 = global read "Global Variables.vi" "Send Count"() -> (→"Send Count":u64)
        n203 = global read "Global Variables.vi" "current run no."() -> (→"Current Run No.":u8)
        n204 = Divide(x=w108, y=i8 78) -> (x/y=w106:dbl)
        n205 = Multiply(x=w106, y=w105) -> (x*y=→"Value [mmHg]" →"Vacuum Force [mmHg]  2":dbl)
        n206 = global read "Global Variables.vi" "assign pt out of bound"() -> (→"Asgn Pt Out of Bound":bool)
        n207 = global read "Global Variables.vi" "tracking timer"() -> (w120:i32)
        n208 = global read "Global Variables.vi" "state changing"() -> (→"State changing":bool)
        n209 = global read "Global Variables.vi" "state flag array"() -> (→"State Flag Array":bool[])
        n210 = Divide(x=w120, y=10) -> (x/y=→"Timer":dbl)
        n211 = flat-sequence {
          frame #0 {
            w147 = sgl[] [0.0, 0.0]  # RCMy
            w146 = sgl[] [0.0, 0.0]  # RCMz
            w148 = sgl[] [0.0, 0.0]  # RCMx
            # "3D Visualization"
            n212 = disable-structure shown="Disabled" {
              disable-tunnel: [w157 _] -> w136
              frame Disabled {
                n213 = global read "Global Variables.vi" "xPC"() -> (w155:dbl[])
                n214 = global read "Global Variables.vi" "yPC"() -> (w154:dbl[])
                n215 = global read "Global Variables.vi" "zPC"() -> (w153:dbl[])
                n216 = call-poly <vilib>:"Plot Helper.vi"("Plot ID"=2, "z vector"=w153, "y vector"=w154, "x vector"=w155) -> ("3D Plot lvclass Array out"=w162:refnum<class "3D Plot Datatype.lvclass">[])  [unwired: 2 in, 5 out]
                n217 = global read "Global Variables.vi" "xACh"() -> (w160:dbl[])
                n218 = global read "Global Variables.vi" "yACh"() -> (w159:dbl[])
                n219 = global read "Global Variables.vi" "zACh"() -> (w158:dbl[])
                n220 = call-poly <vilib>:"Plot Helper.vi"("Plot ID"=3, "z vector"=w158, "y vector"=w159, "x vector"=w160, "3D Plot lvclass Array in"=w162) -> ("3D Plot lvclass Array out"=w157:refnum<class "3D Plot Datatype.lvclass">[])  [unwired: 1 in, 5 out]
              }
              frame Enabled {
              }
            }
            n221 = local read "Tip out Posit"() -> (w140:dbl[])
            n222 = call "Vis Interpolate Points.vi"("Tip out Posit"=w140) -> ("Z"=w137:dbl[], "Y"=w138:dbl[], "X"=w139:dbl[])  [unwired: 4 in]
            n223 = call-poly <vilib>:"Plot Helper.vi"("Plot ID"=1, "z vector"=w137, "y vector"=w138, "x vector"=w139, "3D Plot lvclass Array in"=w136) -> ("3D Plot lvclass Array out"=w130:refnum<class "3D Plot Datatype.lvclass">[])  [unwired: 1 in, 5 out]
            n224 = global read "Global Variables.vi" "xTraj"() -> (w131:dbl[])
            n225 = global read "Global Variables.vi" "yTraj"() -> (w132:dbl[])
            n226 = global read "Global Variables.vi" "zTraj"() -> (w133:dbl[])
            n227 = call-poly <vilib>:"Plot Helper.vi"("Plot ID"=4, "z vector"=w133, "y vector"=w132, "x vector"=w131, "3D Plot lvclass Array in"=w130) -> ("3D Plot lvclass Array out"=w128:refnum<class "3D Plot Datatype.lvclass">[])  [unwired: 1 in, 5 out]
            n228 = disable-structure shown="Disabled" {
              disable-tunnel: w128 -> [w164 w169]
              disable-tunnel: [w163 w169] -> w127
              frame Disabled {
                n229 = global read "Global Variables.vi" "xIris"() -> (w168:dbl[])
                n230 = global read "Global Variables.vi" "yIris"() -> (w167:dbl[])
                n231 = global read "Global Variables.vi" "zIris"() -> (w166:dbl[])
                n232 = call-poly <vilib>:"Plot Helper.vi"("Plot ID"=6, "z vector"=w166, "y vector"=w167, "x vector"=w168, "3D Plot lvclass Array in"=w164) -> ("3D Plot lvclass Array out"=w163:refnum<class "3D Plot Datatype.lvclass">[])  [unwired: 1 in, 5 out]
              }
              frame Enabled {
              }
            }
            n233 = Index Array(array=w140) -> (element #1=w151:dbl, element #2=w150:dbl, element #3=w149:dbl)  [unwired: 3 in]
            n234 = Build Array (concatenate)(w148, w151) -> (w143:dbl[])
            n235 = Build Array (concatenate)(w147, w150) -> (w142:dbl[])
            n236 = Build Array (concatenate)(w146, w149) -> (w141:dbl[])
            n237 = call-poly <vilib>:"Plot Helper.vi"("Plot ID"=5, "z vector"=w141, "y vector"=w142, "x vector"=w143, "3D Plot lvclass Array in"=w127) -> ("3D Plot lvclass Array out"=w134:refnum<class "3D Plot Datatype.lvclass">[])  [unwired: 1 in, 5 out]
            n238 = call-poly <vilib>:"Plot Helper.vi"("Plot ID"=6, "z vector"=w146, "y vector"=w147, "x vector"=w148, "3D Plot lvclass Array in"=w134) -> ("3D Plot lvclass Array out"=→"Robot XYZ":refnum<class "3D Plot Datatype.lvclass">[])  [unwired: 1 in, 5 out]
          }
        }
        n239 = local read "Current System State"() -> (w116:T2)
        n240 = disable-structure shown="Disabled" {
          disable-tunnel: w118 -> [w173 _]
          disable-tunnel: [w172 _] -> w117
          disable-tunnel: w116 -> [w171 _]
          frame Disabled {
            # "Disable write to mitigate finished late"
            n241 = local read item#-1() -> (w170)
            n242 = call "WriteLog.vi"("Online Eye Model"=w170, "Current System State"=w171, "File In"=w173) -> ("File Out"=w172:refnum<file>)  [unwired: 8 in]
          }
          frame Enabled {
          }
        }
        n243 = local read "Program Stop"() -> (w125:bool)
      }
      n244 = while {
        tunnel: w36 -> [w55]
        stop <- w56 stop-if-true
        # "Robot Communication Loop (100 Hz)"
        n245 = Wait (ms)(milliseconds to wait=u32 1) -> ()  [unwired: 1 out]
        n246 = global read "Global Variables.vi" "L1 to L4 cmd Posit"() -> (w42:dbl[])
        n247 = global read "Global Variables.vi" "Stage cmd Posit"() -> (w51:dbl[])
        n248 = global read "Global Variables.vi" "L5 M/S cmd"() -> (w44:dbl)
        n249 = call "MS IRISS V2.vi"("Stage Cmd Posit"=w51, "L5 cmd Posit"=w44, "Joint Cmd Posit"=w42, "ArmID"=w55) -> ("Stage Out Posit"=w50:dbl[], "L5 Out Posit"=w45:dbl, "Joint Out Posit"=w43:dbl[], "Connection Status"=→"Status":bool, "Receive Count"=w52:u64, "Send Count"=w53:u64)  [unwired: 2 in]
        n250 = global write "Global Variables.vi" "L1 to L4 out Posit"(w43) -> ()
        n251 = global write "Global Variables.vi" "L5 out Posit"(w45) -> ()
        n252 = global write "Global Variables.vi" "Stage out Posit"(w50) -> ()
        n253 = global write "Global Variables.vi" "Receive Count"(w52) -> ()
        n254 = global write "Global Variables.vi" "Send Count"(w53) -> ()
        n255 = Index Array(array=w43, index=2) -> (element=w48:dbl)
        n256 = Greater?(x=w48, y=0.05) -> (0:w47:bool)
        n257 = global write "Global Variables.vi" "irrigate"(w47) -> ()
        n258 = local read "Program Stop"() -> (w56:bool)
      }
    }
    frame #3 {
      # "Reset Flags"
      n259 = disable-structure shown="Disabled" {
        disable-tunnel: w317 -> [w318 _]
        frame Disabled {
          n260 = Close File(refnum=w318) -> ()  [unwired: 1 in, 2 out]
        }
        frame Enabled {
        }
      }
      n261 = global write "Global Variables.vi" "irrigate"(FALSE ("irrigate")) -> ()
    }
    frame #4 {
      # "Close Application"
      n262 = global read "Global Variables.vi" "armID"() -> (w319:i32)
      n263 = dll-call lib="D:/Kevin/IRISS V2 dev/Host Demo/Functions/EyeRobotDLL.dll" fn="CloseRobot" label="Close"("id"=w319) -> ()  [unwired: 5 in, 2 out]
    }
  }
